vi "Load Becker-Hickl File Header.vi"(8 "Error In":errorcluster, 11 "File Path Control":path) -> (0 "Error Out":errorcluster, 2 "B& H File Header":T1 {"Header Valid" format="%.0x"; "# Data Blocks" format="%.0x"; "Revision" format="%.0b"}, 3 "File Path out":path)   [LabVIEW 2021, in "Becker-Hickl Files.lvlib"]
uses:
  Becker-Hickl Files.lvlib
  Becker-Hickl File Header Structure.ctl
  Becker-Hickl Read Single I16.vi
  Becker-Hickl Read Single I32.vi
  Becker-Hickl Read Single U16.vi
  Becker-Hickl Read Single U32.vi
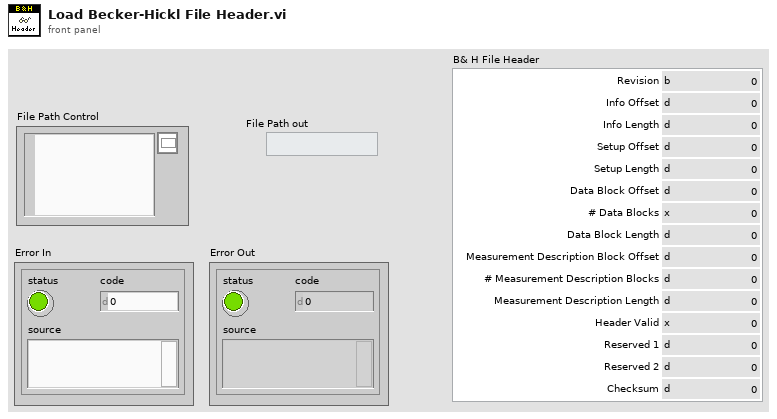
[diagram p1: front panel]
types:
  T1 = typedef "Becker-Hickl Files.lvlib/Becker-Hickl File Header Structure.ctl" = cluster{"Revision":i16, "Info Offset":i32, "Info Length":i16, "Setup Offset":i32, "Setup Length":i16, "Data Block Offset":i32, "# Data Blocks":i16, "Data Block Length":i32, "Measurement Description Block Offset":i32, "# Measurement Description Blocks":i16, "Measurement Description Length":i16, "Header Valid":u16, "Reserved 1":u32, "Reserved 2":u16, "Checksum":u16}
  T2 = enum16{"open", "replace", "create", "open or create", "replace or create", "replace or create with confirmation"}
  T3 = enum16{"revision", "info_offs", "info_length", "setup_offs", "setup_length", "data_block_offs", "no_of_data_blocks", "data_block_length", "meas_desc_block_offs", "no_of_meas_desc_blocks", "meas_desc_block_length", "header_valid", "reserved1", "reserved2", "chksum"}
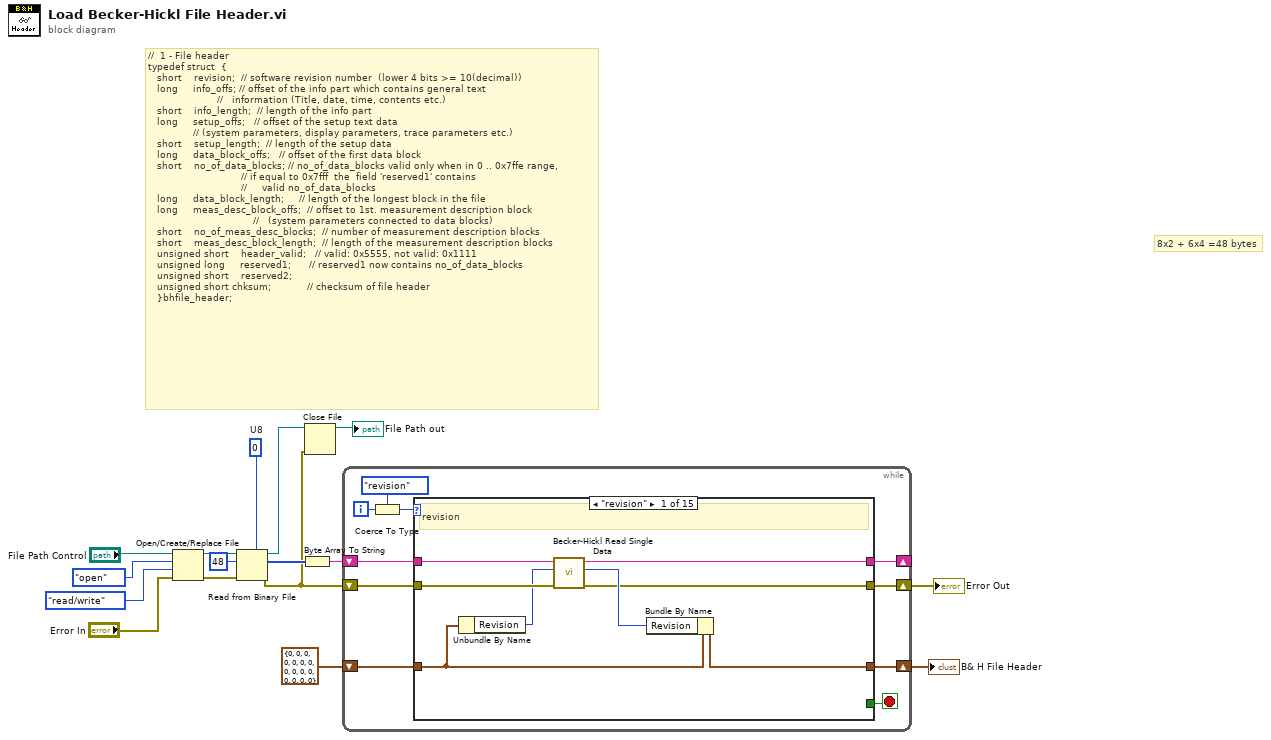
[diagram p0: block diagram]
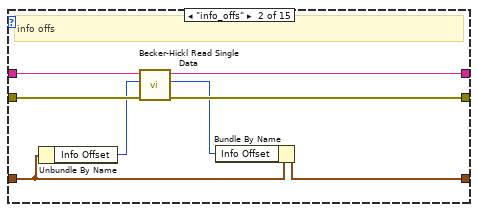
[diagram p2: hidden frame]
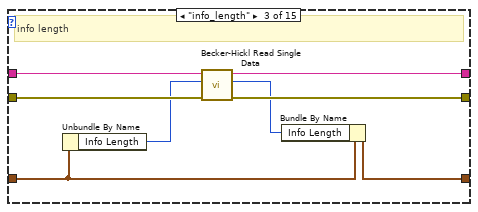
[diagram p3: hidden frame]
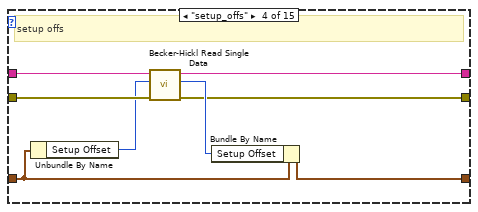
[diagram p4: hidden frame]
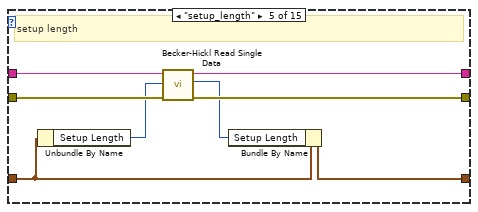
[diagram p5: hidden frame]
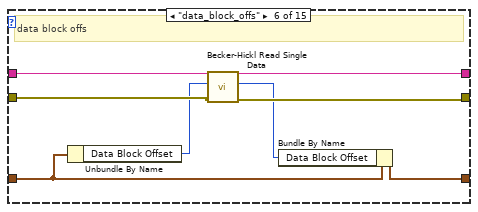
[diagram p6: hidden frame]
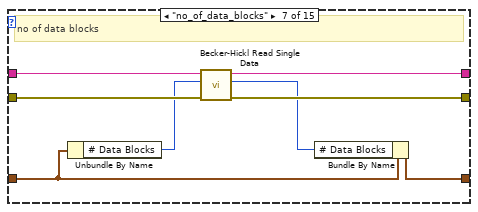
[diagram p7: hidden frame]
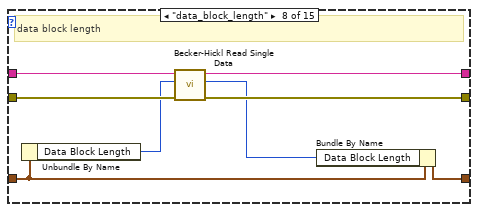
[diagram p8: hidden frame]
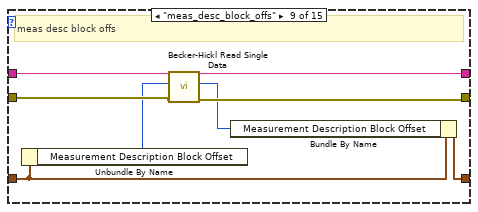
[diagram p9: hidden frame]
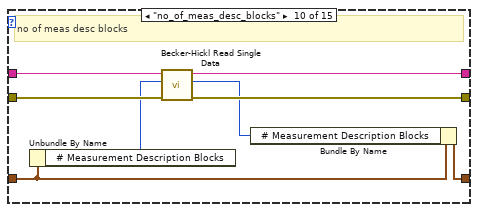
[diagram p10: hidden frame]
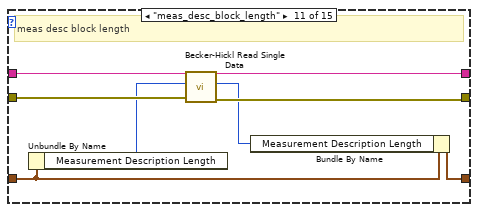
[diagram p11: hidden frame]
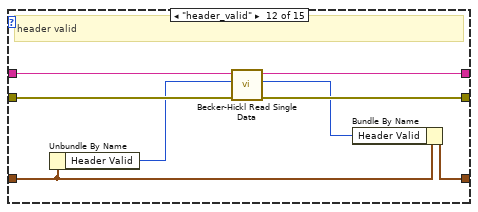
[diagram p12: hidden frame]
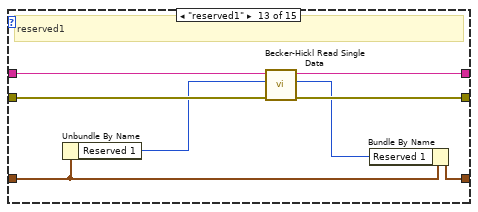
[diagram p13: hidden frame]
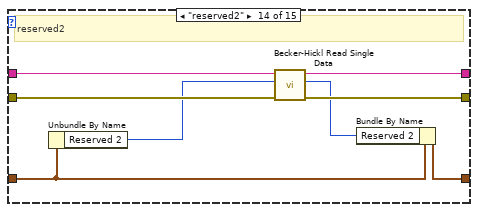
[diagram p14: hidden frame]
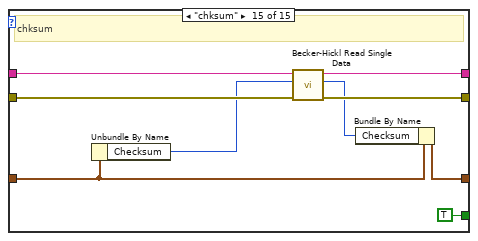
[diagram p15: hidden frame]
diagram:
  w10 = u8 0  # U8
  # "8x2 + 6x4 =48 bytes"
  # "//  1 - File header\ntypedef struct  {\n   short    revision;  // software revision number  (lower 4 bits >= 10(decimal))\n   long     info_offs; // offset of the info part which contains general text \n                       //   information (Title, date, time, contents etc.)\n   short    info_length;  // length of the info part\n   long     setup_offs;   // offset of the setup text data \n               // (system parameters, display parameters, trace parameters etc.)\n   short    setup_length;  // length of the setup data\n   long     data_block_offs;   // offset of the first data block \n   short    no_of_data_blocks; // no_of_data_blocks valid only when in 0 .. 0x7ffe range,\n                               // if equal to 0x7fff  the  field 'reserved1' contains \n                               //     valid no_of_data_blocks\n   long     data_block_length;     // length of the longest block in the file\n   long     meas_desc_block_offs;  // offset to 1st. measurement description block \n                                   //   (system parameters connected to data blocks)\n   short    no_of_meas_desc_blocks;  // number of measurement description blocks\n   short    meas_desc_block_length;  // length of the measurement description blocks\n   unsigned short    header_valid;   // valid: 0x5555, not valid: 0x1111\n   unsigned long     reserved1;      // reserved1 now contains no_of_data_blocks\n   unsigned short    reserved2;\n   unsigned short chksum;            // checksum of file header\n   }bhfile_header;"
  n1 = Open/Create/Replace File(file path (use dialog)="File Path Control", error in="Error In", operation (0:open)=T2."open", access (0:read/write)=enum16{"read/write", "read-only", "write-only"}."read/write") -> (refnum out=w12:refnum<file>, error out=w11:errorcluster)  [unwired: 2 in, 1 out]
  n2 = Read from Binary File(5:w10, 8:w11, 10:48 ("count (1)"), 11:w12) -> (0:w3:errorcluster, 2:w8:u8[], 3:w5:refnum<file>)  [unwired: 2 in, 1 out]
  n3 = Byte Array To String(unsigned byte array=w8) -> (string=w2:string)
  n4 = Close File(refnum=w5, error in=w3) -> (path=→"File Path out":path)  [unwired: 1 out]
  n5 = while {
    shift-right: [w21] -> _
    shift-left: w2 -> [w25]
    shift-right: [w23] -> w6
    shift-left: T1 {"Revision"=0, "Info Offset"=0, "Info Length"=0, "Setup Offset"=0, "Setup Length"=0, "Data Block Offset"=0, "# Data Blocks"=0, "Data Block Length"=0, "Measurement Description Block Offset"=0, "# Measurement Description Blocks"=0, "Measurement Description Length"=0, "Header Valid"=0, "Reserved 1"=0, "Reserved 2"=0, "Checksum"=0} -> [w24]
    shift-right: [w19] -> w1
    shift-left: w3 -> [w20]
    i -> [w26]
    stop <- w22 stop-if-true
    n6 = Coerce To Type(0:w26, 1:T3."revision") -> (2:w18:T3)
    n7 = case shown="\"revision\"" w18 {
      tunnel: w25 -> [w33 w41 w49 w58 w65 w73 w81 w89 w97 w105 w113 w121 w129 w137 w145]
      tunnel: w24 -> [w28 w36 w44 w52 w60 w68 w76 w84 w92 w100 w108 w116 w124 w132 w140]
      tunnel: [w34 w42 w50 w57 w66 w74 w82 w90 w98 w106 w114 w122 w130 w138 w147] -> w23
      tunnel: [_ _ _ _ _ _ _ _ _ _ _ _ _ _ TRUE] -> w22
      tunnel: [w32 w40 w46 w56 w64 w71 w80 w86 w96 w103 w111 w119 w127 w135 w143] -> w21
      tunnel: w20 -> [w30 w39 w48 w54 w63 w72 w79 w88 w95 w104 w112 w120 w128 w136 w144]
      tunnel: [w29 w38 w47 w53 w62 w70 w78 w87 w94 w102 w110 w118 w126 w134 w142] -> w19
      frame "revision" {
        # "revision"
        n8 = Unbundle By Name(w28) -> ("Revision"=w27:i16)
        n9 = call-poly "Becker-Hickl Read Single Data.vi"("Error In"=w30, "Default"=w27, "Bytes in"=w33) -> ("Error Out"=w29:errorcluster, "I16"=w31:i16, "Bytes out"=w32:string)  [unwired: 6 in]
        n10 = Bundle By Name(cluster=w28, "Revision"=w31) -> (w34:T1)
      }
      frame "info_offs" {
        # "info offs"
        n11 = Unbundle By Name(w36) -> ("Info Offset"=w35:i32)
        n12 = call-poly "Becker-Hickl Read Single Data.vi"("Error In"=w39, "Default"=w35, "Bytes in"=w41) -> ("Error Out"=w38:errorcluster, "I32"=w37:i32, "Bytes out"=w40:string)  [unwired: 6 in]
        n13 = Bundle By Name(cluster=w36, "Info Offset"=w37) -> (w42:T1)
      }
      frame "info_length" {
        # "info length"
        n14 = Unbundle By Name(w44) -> ("Info Length"=w43:i16)
        n15 = call-poly "Becker-Hickl Read Single Data.vi"("Error In"=w48, "Default"=w43, "Bytes in"=w49) -> ("Error Out"=w47:errorcluster, "I16"=w45:i16, "Bytes out"=w46:string)  [unwired: 6 in]
        n16 = Bundle By Name(cluster=w44, "Info Length"=w45) -> (w50:T1)
      }
      frame "setup_offs" {
        # "setup offs"
        n17 = Unbundle By Name(w52) -> ("Setup Offset"=w51:i32)
        n18 = call-poly "Becker-Hickl Read Single Data.vi"("Error In"=w54, "Default"=w51, "Bytes in"=w58) -> ("Error Out"=w53:errorcluster, "I32"=w55:i32, "Bytes out"=w56:string)  [unwired: 6 in]
        n19 = Bundle By Name(cluster=w52, "Setup Offset"=w55) -> (w57:T1)
      }
      frame "setup_length" {
        # "setup length"
        n20 = Unbundle By Name(w60) -> ("Setup Length"=w59:i16)
        n21 = call-poly "Becker-Hickl Read Single Data.vi"("Error In"=w63, "Default"=w59, "Bytes in"=w65) -> ("Error Out"=w62:errorcluster, "I16"=w61:i16, "Bytes out"=w64:string)  [unwired: 6 in]
        n22 = Bundle By Name(cluster=w60, "Setup Length"=w61) -> (w66:T1)
      }
      frame "data_block_offs" {
        # "data block offs"
        n23 = Unbundle By Name(w68) -> ("Data Block Offset"=w67:i32)
        n24 = call-poly "Becker-Hickl Read Single Data.vi"("Error In"=w72, "Default"=w67, "Bytes in"=w73) -> ("Error Out"=w70:errorcluster, "I32"=w69:i32, "Bytes out"=w71:string)  [unwired: 6 in]
        n25 = Bundle By Name(cluster=w68, "Data Block Offset"=w69) -> (w74:T1)
      }
      frame "no_of_data_blocks" {
        # "no of data blocks"
        n26 = Unbundle By Name(w76) -> ("# Data Blocks"=w75:i16)
        n27 = call-poly "Becker-Hickl Read Single Data.vi"("Error In"=w79, "Default"=w75, "Bytes in"=w81) -> ("Error Out"=w78:errorcluster, "I16"=w77:i16, "Bytes out"=w80:string)  [unwired: 6 in]
        n28 = Bundle By Name(cluster=w76, "# Data Blocks"=w77) -> (w82:T1)
      }
      frame "data_block_length" {
        # "data block length"
        n29 = Unbundle By Name(w84) -> ("Data Block Length"=w83:i32)
        n30 = call-poly "Becker-Hickl Read Single Data.vi"("Error In"=w88, "Default"=w83, "Bytes in"=w89) -> ("Error Out"=w87:errorcluster, "I32"=w85:i32, "Bytes out"=w86:string)  [unwired: 6 in]
        n31 = Bundle By Name(cluster=w84, "Data Block Length"=w85) -> (w90:T1)
      }
      frame "meas_desc_block_offs" {
        # "meas desc block offs"
        n32 = Unbundle By Name(w92) -> ("Measurement Description Block Offset"=w91:i32)
        n33 = call-poly "Becker-Hickl Read Single Data.vi"("Error In"=w95, "Default"=w91, "Bytes in"=w97) -> ("Error Out"=w94:errorcluster, "I32"=w93:i32, "Bytes out"=w96:string)  [unwired: 6 in]
        n34 = Bundle By Name(cluster=w92, "Measurement Description Block Offset"=w93) -> (w98:T1)
      }
      frame "no_of_meas_desc_blocks" {
        # "no of meas desc blocks"
        n35 = Unbundle By Name(w100) -> ("# Measurement Description Blocks"=w99:i16)
        n36 = call-poly "Becker-Hickl Read Single Data.vi"("Error In"=w104, "Default"=w99, "Bytes in"=w105) -> ("Error Out"=w102:errorcluster, "I16"=w101:i16, "Bytes out"=w103:string)  [unwired: 6 in]
        n37 = Bundle By Name(cluster=w100, "# Measurement Description Blocks"=w101) -> (w106:T1)
      }
      frame "meas_desc_block_length" {
        # "meas desc block length"
        n38 = Unbundle By Name(w108) -> ("Measurement Description Length"=w107:i16)
        n39 = call-poly "Becker-Hickl Read Single Data.vi"("Error In"=w112, "Default"=w107, "Bytes in"=w113) -> ("Error Out"=w110:errorcluster, "I16"=w109:i16, "Bytes out"=w111:string)  [unwired: 6 in]
        n40 = Bundle By Name(cluster=w108, "Measurement Description Length"=w109) -> (w114:T1)
      }
      frame "header_valid" {
        # "header valid"
        n41 = Unbundle By Name(w116) -> ("Header Valid"=w115:u16)
        n42 = call-poly "Becker-Hickl Read Single Data.vi"("Error In"=w120, "Default"=w115, "Bytes in"=w121) -> ("Error Out"=w118:errorcluster, "U16"=w117:u16, "Bytes out"=w119:string)  [unwired: 6 in]
        n43 = Bundle By Name(cluster=w116, "Header Valid"=w117) -> (w122:T1)
      }
      frame "reserved1" {
        # "reserved1"
        n44 = Unbundle By Name(w124) -> ("Reserved 1"=w123:u32)
        n45 = call-poly "Becker-Hickl Read Single Data.vi"("Error In"=w128, "Default"=w123, "Bytes in"=w129) -> ("Error Out"=w126:errorcluster, "U32"=w125:u32, "Bytes out"=w127:string)  [unwired: 6 in]
        n46 = Bundle By Name(cluster=w124, "Reserved 1"=w125) -> (w130:T1)
      }
      frame "reserved2" {
        # "reserved2"
        n47 = Unbundle By Name(w132) -> ("Reserved 2"=w131:u16)
        n48 = call-poly "Becker-Hickl Read Single Data.vi"("Error In"=w136, "Default"=w131, "Bytes in"=w137) -> ("Error Out"=w134:errorcluster, "U16"=w133:u16, "Bytes out"=w135:string)  [unwired: 6 in]
        n49 = Bundle By Name(cluster=w132, "Reserved 2"=w133) -> (w138:T1)
      }
      frame "chksum" {
        # "chksum"
        n50 = Unbundle By Name(w140) -> ("Checksum"=w139:u16)
        n51 = call-poly "Becker-Hickl Read Single Data.vi"("Error In"=w144, "Default"=w139, "Bytes in"=w145) -> ("Error Out"=w142:errorcluster, "U16"=w141:u16, "Bytes out"=w143:string)  [unwired: 6 in]
        n52 = Bundle By Name(cluster=w140, "Checksum"=w141) -> (w147:T1)
      }
    }
  }
  "Error Out" <- w1
  "B& H File Header" <- w6
